vi "Host Image Acquisition Loop.vi"(8 "error in":errorcluster, 11 "Image Reference":refnum<vi>) -> (0 "error out":errorcluster)   [LabVIEW 2013]
doc: "Loop handles the image acquisition communication to FPGA.\nInitialize - Queues up the intialize states\n\nExit"
uses:
  Host Image Acquisition Module Enum.ctl
  Message Passing/MsgQ Loops enum.ctl
  Image Acquisition Settings FG Enum.ctl
  System Status/Status FG Enum.ctl
  Globals/Simulation Settings Global.vi
  Common/State Machines/State Machine Lib.lvlib
  Message Passing/Main MsgQ.lvlib
panel:
  out "State":string
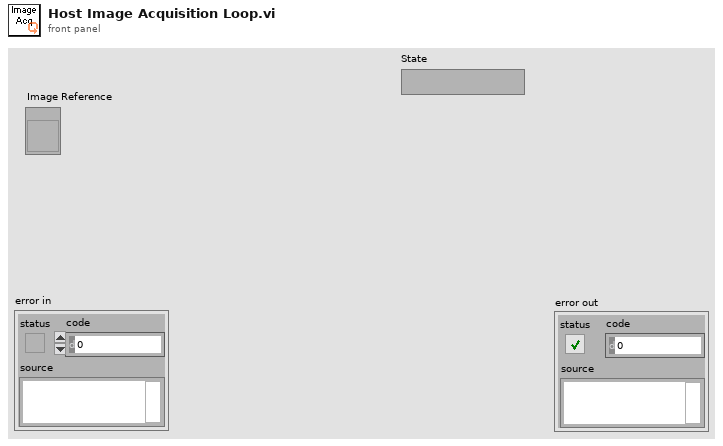
[diagram p1: front panel]
types:
  T1 = typedef "State Machine Lib.lvlib/STATE cluster.ctl" = cluster{"State":string, "Parameters":variant}
  T2 = typedef "Host Image Acquisition Module Enum.ctl" = enum16{"Open FPGA", "Initialize DMA FIFO", "Load Sim Images", "Initialize Acquisition", "Update Sector Parameters", "Start Acquisition", "Aquire Image", "Read Averages", "Cancel Acquisition", "Close FPGA"}
  T3 = typedef "Main MsgQ.lvlib/MsgQ Loops enum.ctl" = enum16{"User Interface", "Image Acq"}
  T4 = typedef "Image Acquisition Settings FG Enum.ctl" = enum16{"Read", "Write"}
  T5 = typedef "Status FG Enum.ctl" = enum16{"Reset", "Read", "Write"}
  T6 = typedef "Simulation Settings Cluster.ctl" = cluster{"Sim Enabled?":bool, "Sim Path":path}
  T7 = typedef "IMAQ Image.ctl" = refnum<image>
  T8 = typedef "Acquisition Settings Cluster.ctl" = cluster{"Image Width":u32, "Image Height":u32, "Frames To Acquire":u32, "Signal Mapping":enum8{"Standard", "Basler 10-tap", "Vosskühler 10-tap"}, "DMA Buffer Size\n(In Images)":u32}
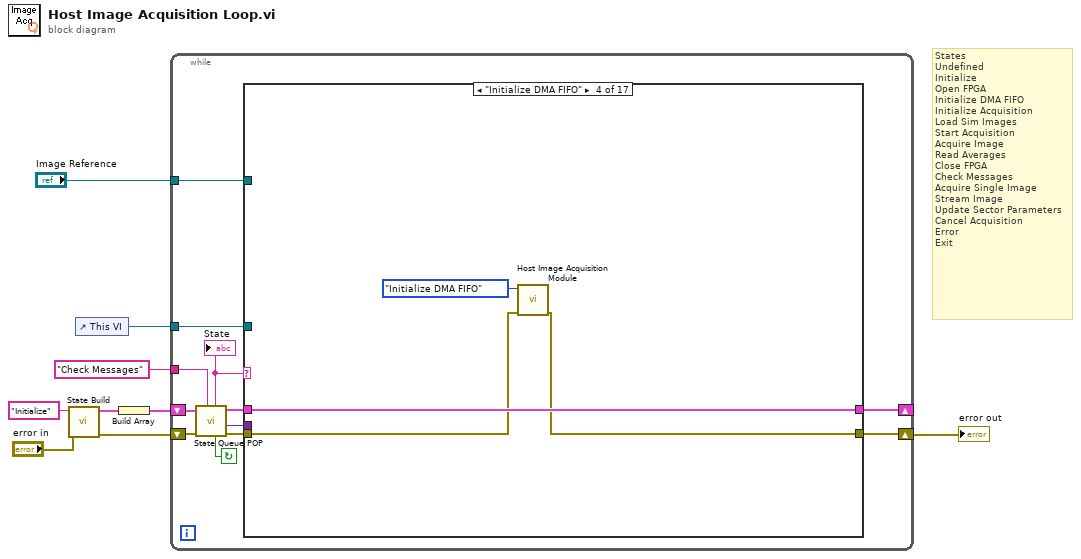
[diagram p0: block diagram]
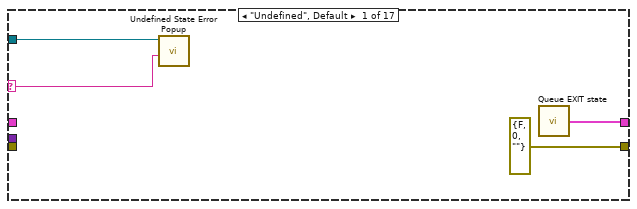
[diagram p2: hidden frame]
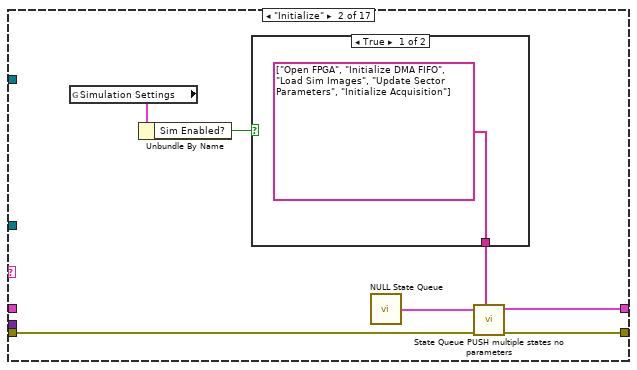
[diagram p3: hidden frame]
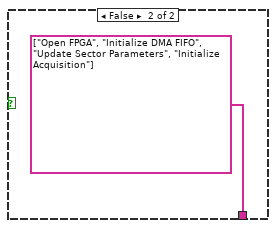
[diagram p4: hidden frame]
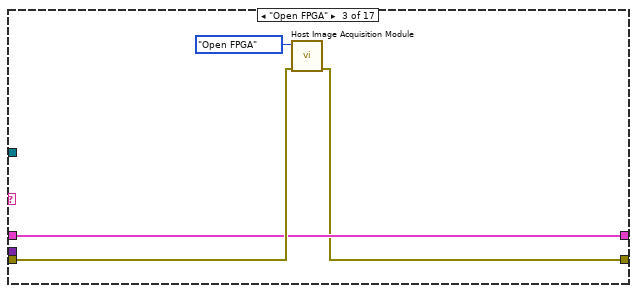
[diagram p5: hidden frame]
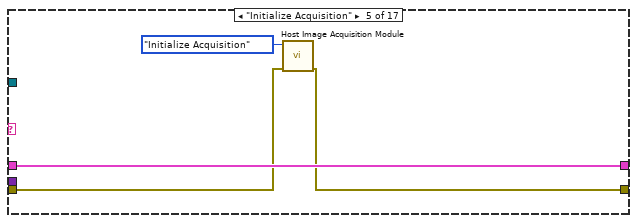
[diagram p6: hidden frame]
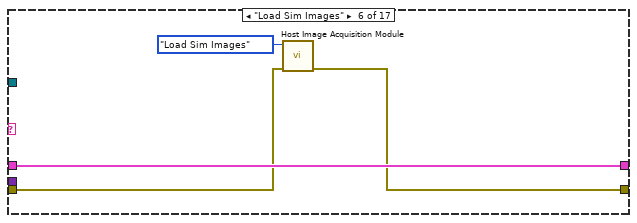
[diagram p7: hidden frame]
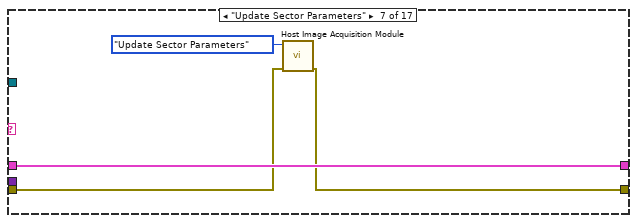
[diagram p8: hidden frame]
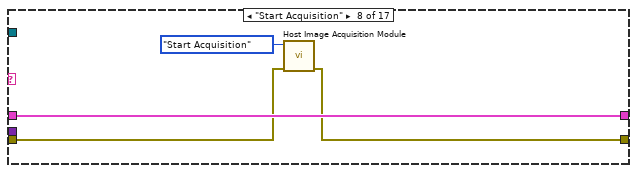
[diagram p9: hidden frame]
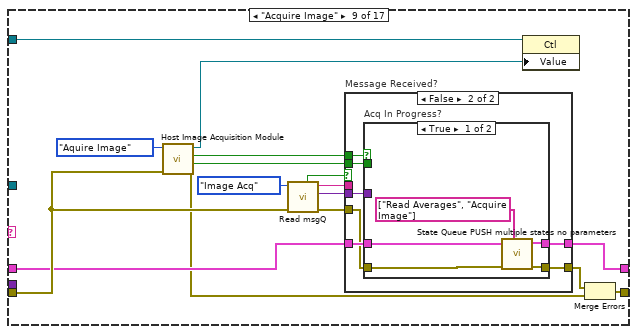
[diagram p10: hidden frame]
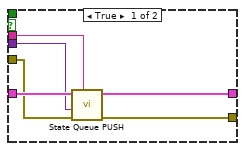
[diagram p11: hidden frame]
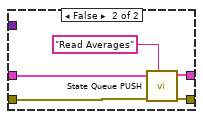
[diagram p12: hidden frame]
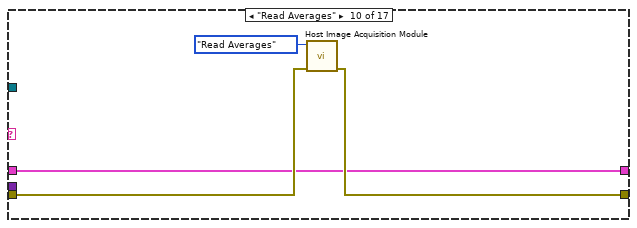
[diagram p13: hidden frame]
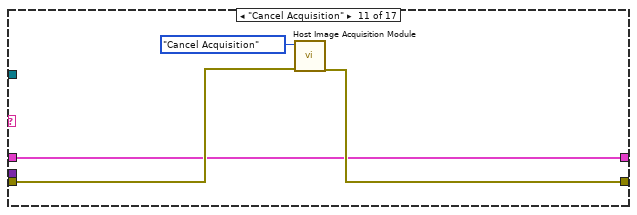
[diagram p14: hidden frame]
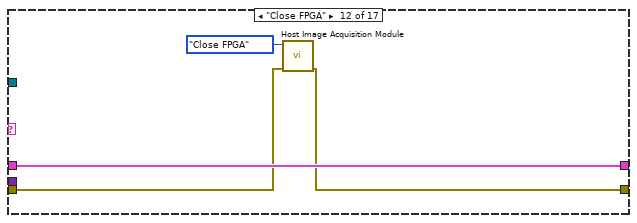
[diagram p15: hidden frame]
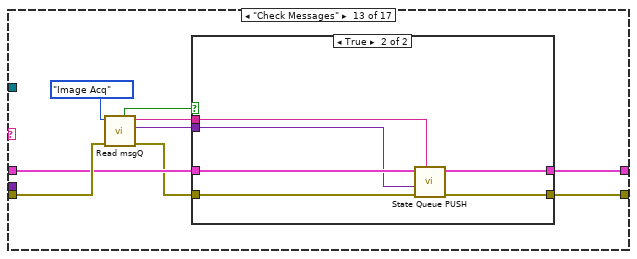
[diagram p16: hidden frame]
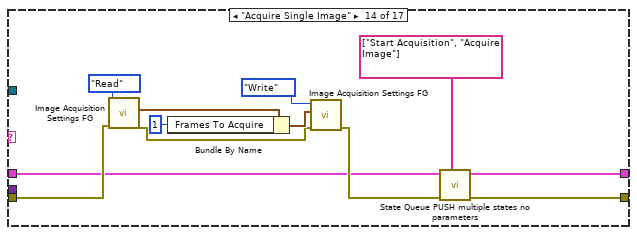
[diagram p18: hidden frame]
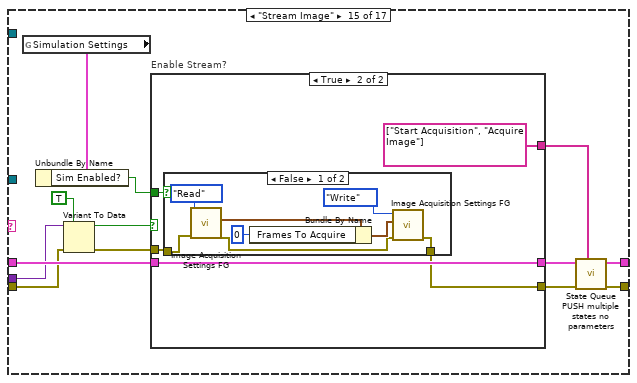
[diagram p19: hidden frame]
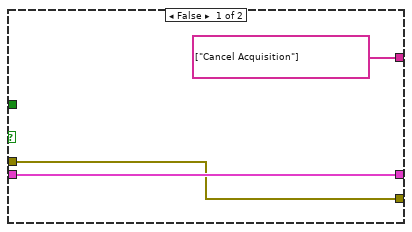
[diagram p20: hidden frame]
diagram:
  # "States\nUndefined\nInitialize\nOpen FPGA\nInitialize DMA FIFO\nInitialize Acquisition\nLoad Sim Images\nStart Acquisition\nAcquire Image\nRead Averages\nClose FPGA\nCheck Messages\nAcquire Single Image\nStream Image\nUpdate Sector Parameters\nCancel Acquisition\nError\nExit"
  n1 = call "State Build.vi"("error in (no error)"="error in", "State"="Initialize") -> ("error out"=w5:errorcluster, "State Out"=w7:T1)  [unwired: 8 in]
  n2 = control-ref of="This VI"() -> (w2:refnum<vi>)
  n3 = Build Array(w7) -> (w6:T1[])
  n4 = while {
    shift-right: [w14] -> _
    shift-left: w6 -> [w21]
    shift-right: [w13] -> w3
    shift-left: w5 -> [w20]
    tunnel: "Check Messages" ("Default state") -> [w18]
    tunnel: w2 -> [w12]
    tunnel: "Image Reference" -> [w11]
    stop <- w19 continue-if-true
    n5 = call "State Queue POP.vi"("Default state"=w18, "error in (no error)"=w20, "State que in"=w21) -> ("error out"=w15:errorcluster, "Parameters"=w10:variant, "State que out"=w16:T1[], "Not Exit?"=w19:bool, "State case out"=w17:string)  [unwired: 4 in]
    "State" <- w17
    n6 = case shown="\"Initialize DMA FIFO\"" w17 {
      selector: w17 -> [w24 _ _ _ _ _ _ _ _ _ _ _ _ _ _ _ _]
      tunnel: w16 -> [_ _ w36 w42 w46 w50 w54 w58 w68 w98 w102 w109 w116 w130 w151 w171 w178]
      tunnel: w15 -> [_ w32 w37 w41 w45 w49 w53 w57 w71 w100 w104 w108 w118 w137 w141 w174 w177]
      tunnel: [w23 w29 w36 w42 w46 w50 w54 w58 w67 w98 w102 w109 w115 w128 w146 w171 w178] -> w14
      tunnel: [errorcluster {"status"=FALSE, "code"=0, "source"=""} ("error out") w28 w35 w40 w44 w47 w52 w56 w64 w99 w103 w107 w114 w127 w144 w172 w177] -> w13
      tunnel: w12 -> [w25 _ _ _ _ _ _ _ _ _ _ _ _ _ _ _ _]
      tunnel: w11 -> [_ _ _ _ _ _ _ _ w63 _ _ _ _ _ _ _ _]
      tunnel: w10 -> [_ _ _ _ _ _ _ _ _ _ _ _ _ _ w150 _ _]
      frame "Undefined", Default {
        n7 = call "Undefined State Error Popup.vi"("String"=w24, "This VI (Caller if unwired)"=w25) -> ()  [unwired: 10 in]
        n8 = call "Queue EXIT state.vi"() -> ("Exit State Q"=w23:T1[])  [unwired: 1 in]
      }
      frame "Initialize" {
        n9 = global read "Simulation Settings Global.vi" "Simulation Settings"() -> (w27:T6)
        n10 = Unbundle By Name(w27) -> ("Sim Enabled?"=w26:bool)
        n11 = case shown="True" w26 {
          tunnel: [string[] ["Open FPGA", "Initialize DMA FIFO", "Load Sim Images", "Update Sector Parameters", "Initialize Acquisition"] ("States to queue") string[] ["Open FPGA", "Initialize DMA FIFO", "Update Sector Parameters", "Initialize Acquisition"] ("States to queue")] -> w30
          frame True {
          }
          frame False {
          }
        }
        n12 = call "NULL State Queue.vi"() -> ("NULL State Queue"=w31:T1[])
        n13 = call "State Queue PUSH multiple states no parameters.vi"("States to queue"=w30, "error in (no error)"=w32, "State que in"=w31) -> ("error out"=w28:errorcluster, "State que out"=w29:T1[])  [unwired: 7 in]
      }
      frame "Open FPGA" {
        n14 = call "Host Image Acquisition Module.vi"("error in"=w37, "Operation"=Host_Image_Acquisition_Module_Enum."Open FPGA") -> ("error out"=w35:errorcluster)  [unwired: 6 in, 3 out]
      }
      frame "Initialize DMA FIFO" {
        n15 = call "Host Image Acquisition Module.vi"("error in"=w41, "Operation"=Host_Image_Acquisition_Module_Enum."Initialize DMA FIFO") -> ("error out"=w40:errorcluster)  [unwired: 6 in, 3 out]
      }
      frame "Initialize Acquisition" {
        n16 = call "Host Image Acquisition Module.vi"("error in"=w45, "Operation"=Host_Image_Acquisition_Module_Enum."Initialize Acquisition") -> ("error out"=w44:errorcluster)  [unwired: 6 in, 3 out]
      }
      frame "Load Sim Images" {
        n17 = call "Host Image Acquisition Module.vi"("error in"=w49, "Operation"=Host_Image_Acquisition_Module_Enum."Load Sim Images") -> ("error out"=w47:errorcluster)  [unwired: 6 in, 3 out]
      }
      frame "Update Sector Parameters" {
        n18 = call "Host Image Acquisition Module.vi"("error in"=w53, "Operation"=Host_Image_Acquisition_Module_Enum."Update Sector Parameters") -> ("error out"=w52:errorcluster)  [unwired: 6 in, 3 out]
      }
      frame "Start Acquisition" {
        n19 = call "Host Image Acquisition Module.vi"("error in"=w57, "Operation"=Host_Image_Acquisition_Module_Enum."Start Acquisition") -> ("error out"=w56:errorcluster)  [unwired: 6 in, 3 out]
      }
      frame "Acquire Image" {
        n20 = call "Host Image Acquisition Module.vi"("error in"=w71, "Operation"=Host_Image_Acquisition_Module_Enum."Aquire Image") -> ("error out"=w65:errorcluster, "Image Acquired"=w59:bool, "Acq In Progress"=w61:bool, "Image"=w62:T7)  [unwired: 6 in]
        n21 = call "Read msgQ.vi"("error in"=w71, "MsgQ enum"=MsgQ_Loops_enum."Image Acq") -> ("error out"=w69:errorcluster, "Message Received Parameters"=w60:variant, "Message Received String"=w70:string, "Message Recieved?"=w72:bool)  [unwired: 6 in]
        n22 = case "Message Received?" shown="False" w72 {
          tunnel: w70 -> [w79 _]
          tunnel: w69 -> [w78 w86]
          tunnel: w68 -> [w80 w87]
          tunnel: [w77 w85] -> w66
          tunnel: [w76 w84] -> w67
          tunnel: w61 -> [_ w83]
          tunnel: w60 -> [w75 w82]
          tunnel: w59 -> [_ w81]
          frame True {
            n23 = call "State Queue PUSH.vi"("State case"=w79, "error in (no error)"=w78, "Parameters"=w75, "State que in"=w80) -> ("error out"=w77:errorcluster, "State que out"=w76:T1[])  [unwired: 6 in]
          }
          frame False {
            n24 = case "Acq In Progress?" shown="True" w83 {
              tunnel: w87 -> [w92 w97]
              tunnel: w86 -> [w89 w94]
              tunnel: [w90 w95] -> w85
              tunnel: [w91 w96] -> w84
              tunnel: w82 -> [_ _]
              tunnel: w81 -> [_ _]
              frame True {
                n25 = call "State Queue PUSH multiple states no parameters.vi"("States to queue"=string[] ["Read Averages", "Acquire Image"], "error in (no error)"=w89, "State que in"=w92) -> ("error out"=w90:errorcluster, "State que out"=w91:T1[])  [unwired: 7 in]
              }
              frame False {
                n26 = call "State Queue PUSH.vi"("State case"="Read Averages", "error in (no error)"=w94, "State que in"=w97) -> ("error out"=w95:errorcluster, "State que out"=w96:T1[])  [unwired: 7 in]
              }
            }
          }
        }
        n27 = property class="Ctl"(reference=w63, "Value"=w62) -> ()  [unwired: 1 in, 2 out]
        n28 = Merge Errors(w66, w65) -> (w64:errorcluster)
      }
      frame "Read Averages" {
        n29 = call "Host Image Acquisition Module.vi"("error in"=w100, "Operation"=Host_Image_Acquisition_Module_Enum."Read Averages") -> ("error out"=w99:errorcluster)  [unwired: 6 in, 3 out]
      }
      frame "Cancel Acquisition" {
        n30 = call "Host Image Acquisition Module.vi"("error in"=w104, "Operation"=Host_Image_Acquisition_Module_Enum."Cancel Acquisition") -> ("error out"=w103:errorcluster)  [unwired: 6 in, 3 out]
      }
      frame "Close FPGA" {
        n31 = call "Host Image Acquisition Module.vi"("error in"=w108, "Operation"=Host_Image_Acquisition_Module_Enum."Close FPGA") -> ("error out"=w107:errorcluster)  [unwired: 6 in, 3 out]
      }
      frame "Check Messages" {
        n32 = call "Read msgQ.vi"("error in"=w118, "MsgQ enum"=MsgQ_Loops_enum."Image Acq") -> ("error out"=w113:errorcluster, "Message Received Parameters"=w110:variant, "Message Received String"=w112:string, "Message Recieved?"=w117:bool)  [unwired: 6 in]
        n33 = case shown="True" w117 {
          tunnel: w116 -> [w120 w126]
          tunnel: [w120 w125] -> w115
          tunnel: [w119 w124] -> w114
          tunnel: w113 -> [w119 w123]
          tunnel: w112 -> [_ w121]
          tunnel: w110 -> [_ w122]
          frame False {
          }
          frame True {
            n34 = call "State Queue PUSH.vi"("State case"=w121, "error in (no error)"=w123, "Parameters"=w122, "State que in"=w126) -> ("error out"=w124:errorcluster, "State que out"=w125:T1[])  [unwired: 6 in]
          }
        }
      }
      frame "Acquire Single Image" {
        n35 = call "Image Acquisition Settings FG.vi"("error in (no error)"=w137, "Operation"=Image_Acquisition_Settings_FG_Enum."Read") -> ("error out"=w132:errorcluster, "Acquisition Settings Out"=w136:T8)  [unwired: 8 in]
        n36 = Bundle By Name(cluster=w136, "Frames To Acquire"=u32 1) -> (w134:T8)
        n37 = call "Image Acquisition Settings FG.vi"("error in (no error)"=w132, "Acquisition Settings In"=w134, "Operation"=Image_Acquisition_Settings_FG_Enum."Write") -> ("error out"=w131:errorcluster)  [unwired: 7 in, 1 out]
        n38 = call "State Queue PUSH multiple states no parameters.vi"("States to queue"=string[] ["Start Acquisition", "Acquire Image"], "error in (no error)"=w131, "State que in"=w130) -> ("error out"=w127:errorcluster, "State que out"=w128:T1[])  [unwired: 7 in]
      }
      frame "Stream Image" {
        n39 = global read "Simulation Settings Global.vi" "Simulation Settings"() -> (w142:T6)
        n40 = Unbundle By Name(w142) -> ("Sim Enabled?"=w139:bool)
        n41 = Variant To Data(error in=w141, type=TRUE, Variant=w150) -> (data=w148:bool, error out=w140:errorcluster)
        n42 = case "Enable Stream?" shown="True" w148 {
          tunnel: w140 -> [w152 w159]
          tunnel: w151 -> [w153 w158]
          tunnel: [w153 w158] -> w147
          tunnel: [w152 w157] -> w145
          tunnel: [string[] ["Cancel Acquisition"] ("States to queue") string[] ["Start Acquisition", "Acquire Image"] ("States to queue")] -> w143
          tunnel: w139 -> [_ w155]
          frame False {
          }
          frame True {
            n43 = case shown="False" w155 {
              tunnel: w159 -> [w166 w168]
              tunnel: [w160 w168] -> w157
              frame False {
                n44 = call "Image Acquisition Settings FG.vi"("error in (no error)"=w166, "Operation"=Image_Acquisition_Settings_FG_Enum."Read") -> ("error out"=w161:errorcluster, "Acquisition Settings Out"=w165:T8)  [unwired: 8 in]
                n45 = Bundle By Name(cluster=w165, "Frames To Acquire"=u32 0) -> (w163:T8)
                n46 = call "Image Acquisition Settings FG.vi"("error in (no error)"=w161, "Acquisition Settings In"=w163, "Operation"=Image_Acquisition_Settings_FG_Enum."Write") -> ("error out"=w160:errorcluster)  [unwired: 7 in, 1 out]
              }
              frame True {
              }
            }
          }
        }
        n47 = call "State Queue PUSH multiple states no parameters.vi"("States to queue"=w143, "error in (no error)"=w145, "State que in"=w147) -> ("error out"=w144:errorcluster, "State que out"=w146:T1[])  [unwired: 7 in]
      }
      frame "Error" {
        n48 = Unbundle By Name(w174) -> ("source"=w175:string)
        n49 = Concatenate Strings("Error: " ("string"), w175) -> (w170:string)
        n50 = call "Status FG.vi"("Status In"=w170, "Operation"=Status_FG_Enum."Write") -> ()  [unwired: 8 in, 2 out]
        n51 = call "Broadcast Exit.vi"("error in"=errorcluster {"status"=FALSE, "code"=0, "source"=""}) -> ("error out"=w172:errorcluster)  [unwired: 10 in]
      }
      frame "Exit" {
      }
    }
  }
  "error out" <- w3
